vi "LinearSystemSim_GetOutput_Single.vi"(9 "Row":i32, 11 "LinearSysemSim":T1) -> (3 "Output":dbl)   [LabVIEW 2019, in "Trajectory_Library.lvlib"]
doc: "Returns an element of the current output of the plant.\n \nInputs:\n - LinearSystemSim -- Data cluster\n - row -- The row to return.\n\nOutputs:\n - Output -- An element of the current output of the plant."
uses:
  Trajectory_Library.lvlib
  LINEAR_SYSTEM_SIM.ctl
  LINEAR_SYSTEM.ctl
  <vilib>/Analysis/Matrix/Datatypes/RealMatrix.ctl
  <vilib>/Analysis/Matrix/NI_Matrix.lvlib
panel:
  # "<States, 1>"
  # "<Outputs, 1>"
  # "<Inputs, 1>"
  # "<Outputs, 1>"
  # "<States,States>"
  # "<States,Inputs>"
  # "<Outputs,States>"
  # "<Outputs,Inputs>"
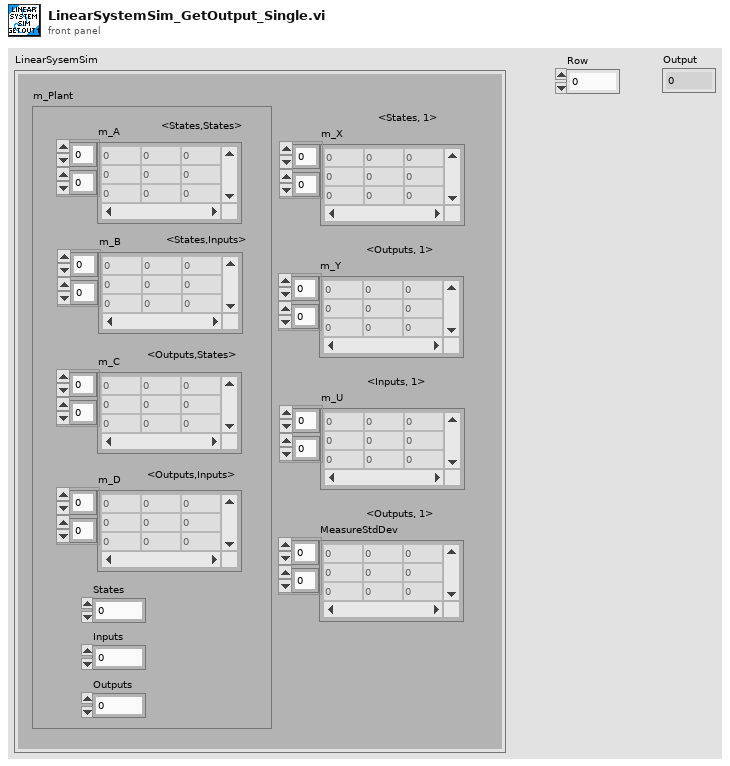
[diagram p1: front panel]
types:
  T1 = typedef "Trajectory_Library.lvlib/LINEAR_SYSTEM_SIM.ctl" = cluster{"m_Plant":T2, "m_X":T3, "m_Y":T3, "m_U":T3, "MeasureStdDev":T3}
  T2 = typedef "Trajectory_Library.lvlib/LINEAR_SYSTEM.ctl" = cluster{"m_A":T3, "m_B":T3, "m_C":T3, "m_D":T3, "States":i32, "Inputs":i32, "Outputs":i32}
  T3 = typedef "NI_Matrix.lvlib/RealMatrix.ctl" = dbl[][]
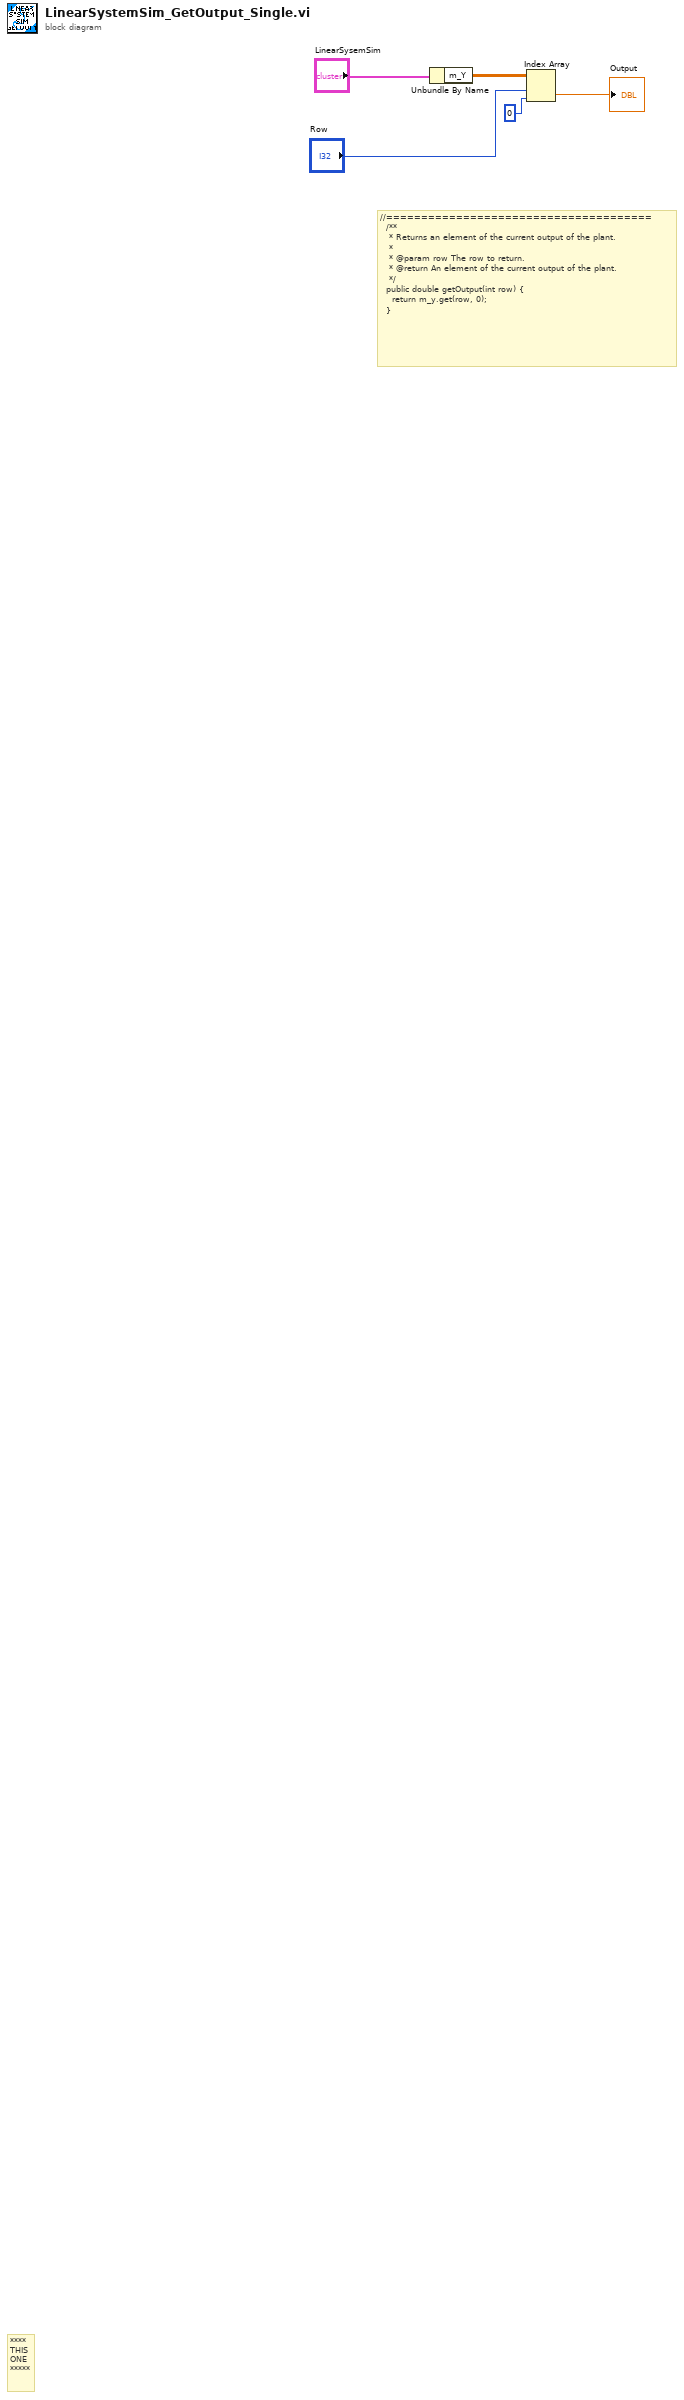
[diagram p0: block diagram]
diagram:
  # "//======================================\n  /**\n   * Returns an element of the current output of the plant.\n   *\n   * @param row The row to return.\n   * @return An element of the current output of the plant.\n   */\n  public double getOutput(int row) {\n    return m_y.get(row, 0);\n  }"
  # "****\nTHIS\nONE\n*****"
  n1 = Unbundle By Name("LinearSysemSim") -> ("m_Y"=w4:T3)
  n2 = Index Array(array=w4, index (row)="Row", index (col)=0) -> (element=→"Output":dbl)
